vi "TestPing.vi"() -> ()   [LabVIEW 2009]
uses:
  Packet.ctl
panel:
  out "error out":errorcluster
  out "Type Good":bool
  out "Data Good":bool
  out "PID Good":bool
  in  "VISA resource name":refnum<visa-resource-name>
  out "PIDReceived":u8
  out "DataReceived":u8[](array[numeric])
  in  "Data":u8[](array[numeric])
  in  "PID":u8
  out "AllGood":bool
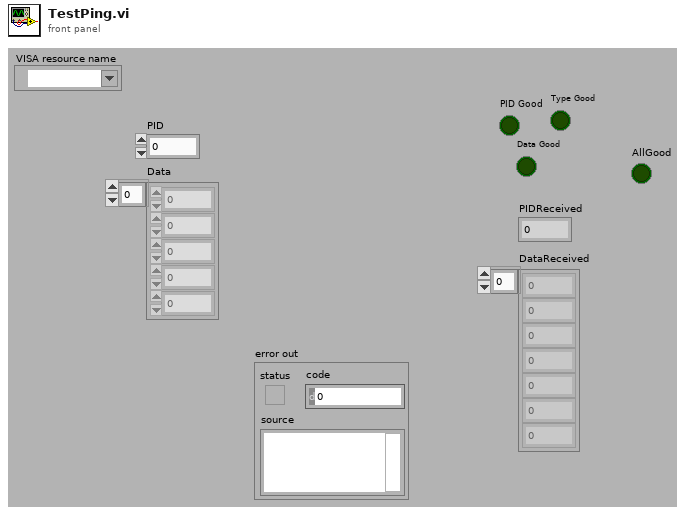
[diagram p1: front panel]
types:
  T1 = typedef "Packet.ctl" = cluster{"Length":u8, "Type":u8, "PID":u8, "Data":u8[], "CRC":u8}
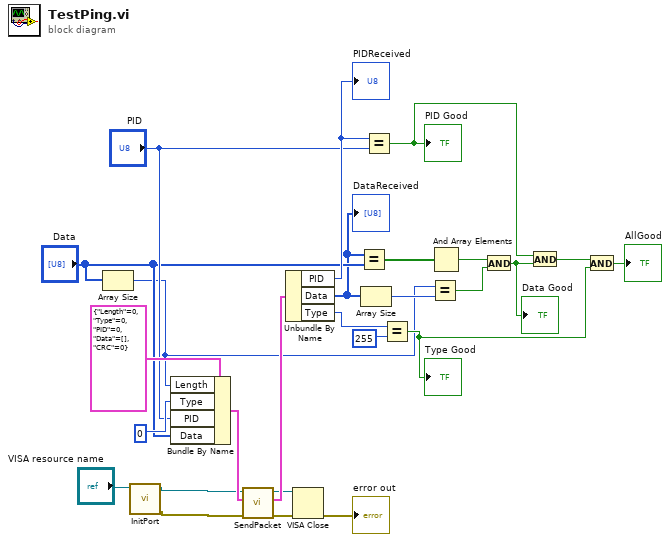
[diagram p0: block diagram]
diagram:
  n1 = Array Size(array="Data") -> (size(s)=w7:i32)
  n2 = call "InitPort.vi"("VISA resource name"="VISA resource name") -> ("error out"=w2:errorcluster, "VISA resource name out"=w3:refnum<visa-resource-name>)  [unwired: 9 in]
  n3 = Bundle By Name(cluster=T1 {"Length"=0, "Type"=0, "PID"=0, "Data"=[], "CRC"=0} ("Transmit"), "Length"=w7, "Type"=u8 0, "PID"="PID", "Data"="Data") -> (w25:T1)
  n4 = call "SendPacket.vi"("error in (no error)"=w2, "Transmit"=w25, "VISA resource name"=w3) -> ("error out"=w10:errorcluster, "Response"=w24:T1, "VISA resource name out"=w12:refnum<visa-resource-name>)  [unwired: 6 in]
  n5 = Unbundle By Name(w24) -> ("PID"=w20:u8, "Data"=w8:u8[], "Type"=w23:u8)
  "DataReceived" <- w8
  "PIDReceived" <- w20
  n6 = VISA Close(VISA resource name=w12, error in (no error)=w10) -> (error out=→"error out":errorcluster)
  n7 = Equal?(x=w8, y="Data") -> (x = y?=w16:bool[])
  n8 = Array Size(array=w8) -> (size(s)=w9:i32)
  n9 = Equal?(x=w20, y="PID") -> (x = y?=w15:bool)
  "PID Good" <- w15
  n10 = Equal?(x=w23, y=u8 255) -> (x = y?=w17:bool)
  "Type Good" <- w17
  n11 = Equal?(x=w7, y=w9) -> (x = y?=w6:bool)
  n12 = And Array Elements(Boolean array=w16) -> (logical AND=w5:bool)
  n13 = And(x=w5, y=w6) -> (x .and. y?=w4:bool)
  "Data Good" <- w4
  n14 = And(x=w15, y=w4) -> (x .and. y?=w14:bool)
  n15 = And(x=w14, y=w17) -> (x .and. y?=→"AllGood":bool)
